vi "test StaticWrite (Func Global).vi"(8 "error in (no error)":errorcluster, 11 "TestCase in":refnum<class "Interface Framework Multiple Objects.lvclass">) -> (0 "error out":errorcluster, 3 "TestCase out":refnum<class "Interface Framework Multiple Objects.lvclass">)   [LabVIEW 2009, in "Interface Framework Multiple Objects.lvclass"]
uses:
  Interface Framework Multiple Objects.lvclass
  Interface Framework Multiple Objects.lvclass/Interface Framework Multiple Objects.ctl
  Numeric Test Object/Interface Implementations/IIntStatic (Func Global)/IIntStatic (Func Global).lvclass
  Numeric Test Object/Numeric Test Object.lvclass
  <vilib>/addons/_JKI Toolkits/VI Tester/TestCase.llb/TestCase.lvclass
  Source/Interfaceable Class/Interfaceable.lvclass
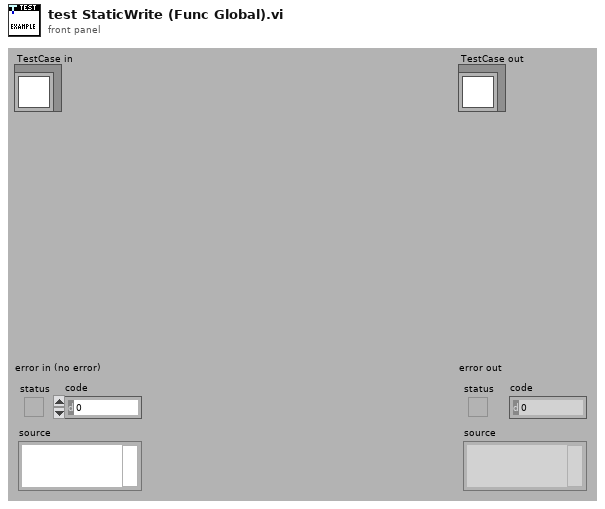
[diagram p1: front panel]
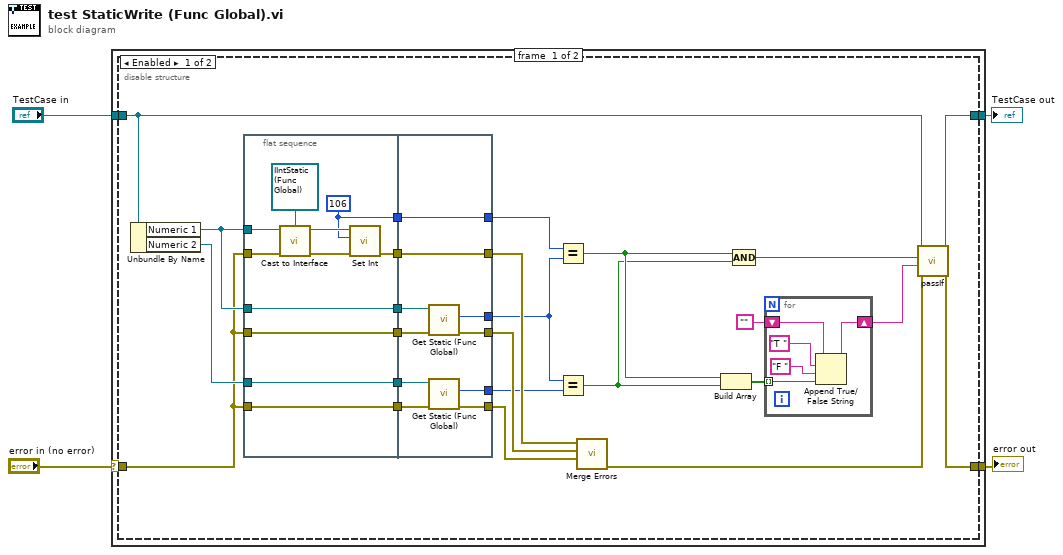
[diagram p0: block diagram]
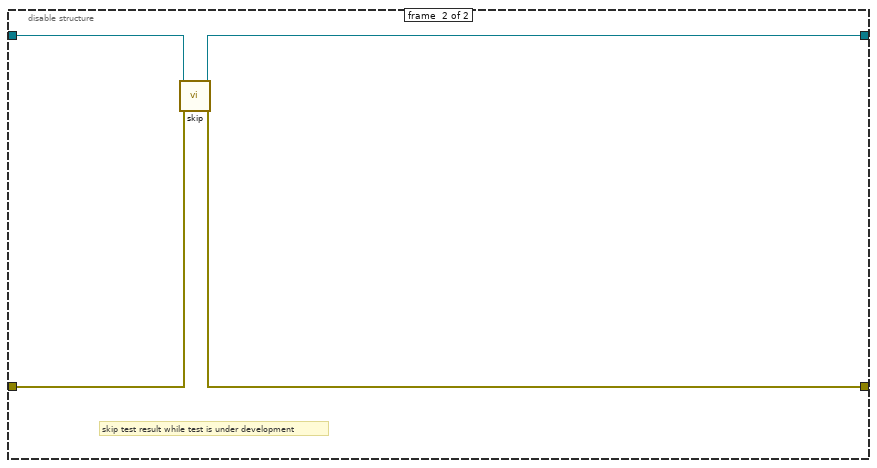
[diagram p2: hidden frame]
diagram:
  n1 = case shown="No Error" "error in (no error)" {
    selector: "error in (no error)" -> [w6 w65]
    tunnel: [w5 w65] -> w3
    tunnel: [w7 w64] -> w1
    tunnel: "TestCase in" -> [w8 w64]
    frame #0 {
      n2 = disable-structure shown="Enabled" {
        disable-tunnel: w8 -> [w31 w63]
        disable-tunnel: [w33 w60] -> w7
        disable-tunnel: w6 -> [w23 w62]
        disable-tunnel: [w32 w61] -> w5
        frame #0 {
          n3 = Unbundle By Name(w31) -> ("Numeric 1"=w29:refnum<class "Numeric Test Object.lvclass">, "Numeric 2"=w30:refnum<class "Numeric Test Object.lvclass">)
          n4 = flat-sequence {
            tunnel: w29 -> [w48]
            tunnel: w30 -> [w41]
            tunnel: w29 -> [w43]
            tunnel: w23 -> [w47]
            tunnel: [w45] -> w28
            tunnel: [w43] -> w27
            tunnel: [w41] -> w26
            tunnel: [w42] -> w25
            tunnel: [w40] -> w24
            tunnel: w23 -> [w40]
            tunnel: w23 -> [w42]
            tunnel: [w39] -> w9
            tunnel: [w51] -> w19
            tunnel: w28 -> [w51]
            tunnel: w27 -> [w59]
            tunnel: w26 -> [w58]
            tunnel: w25 -> [w57]
            tunnel: w24 -> [w56]
            tunnel: [w55] -> w20
            tunnel: [w54] -> w21
            tunnel: [w53] -> w18
            tunnel: [w52] -> w17
            tunnel: [w50] -> w10
            tunnel: w9 -> [w50]
            frame #0 {
              w39 = 106 ("Int")
              n5 = call "Cast to Interface.vi"("Target Interface"=refnum<class "IIntStatic (Func Global).lvclass"> refnum ("IIntByRef.lvclass"), "Interfaceable Object"=w48, "error in (no error)"=w47) -> ("Concrete Interface"=w49:refnum<class "IIntStatic (Func Global).lvclass">, "error out"=w46:errorcluster)  [unwired: 5 in]
              n6 = call-dynamic "Set Int.vi"("error in (no error)"=w46, "Int"=w39, "IIntStatic in"=w49) -> ("error out"=w45:errorcluster)  [unwired: 7 in, 1 out]
            }
            frame #1 {
              n7 = call-dynamic "Get Static (Func Global).vi"("error in (no error)"=w57, "Numeric in"=w59) -> ("error out"=w55:errorcluster, "Int"=w53:i32)  [unwired: 7 in, 1 out]
              n8 = call-dynamic "Get Static (Func Global).vi"("error in (no error)"=w56, "Numeric in"=w58) -> ("error out"=w54:errorcluster, "Int"=w52:i32)  [unwired: 7 in, 1 out]
            }
          }
          n9 = Equal?(x=w10, y=w18) -> (x = y?=w12:bool)
          n10 = Equal?(x=w18, y=w17) -> (x = y?=w11:bool)
          n11 = call <vilib>:"Merge Errors.vi"("error in 3 (no error)"=w21, "error in 2 (no error)"=w20, "error in 1 (no error)"=w19) -> ("error out"=w22:errorcluster)  [unwired: 4 in]
          n12 = Build Array(w12, w11) -> (w15:bool[])
          n13 = Compound Arithmetic op=AND(w12, w11) -> (w14:bool)
          n14 = for {
            tunnel: w15 -> [w38] mode=indexing
            shift-right: [w37] -> w13
            shift-left: "" -> [w34]
            n15 = Append True/False String(1:w38, 2:"F " ("false string"), 3:"T " ("true string"), 4:w34) -> (0:w37:string)
          }
          n16 = call-dynamic "passIf.vi"("error in (no error)"=w22, "message (\"\")"=w13, "pass"=w14, "TestCase in"=w31) -> ("error out"=w32:errorcluster, "TestCase out"=w33:refnum<class "Interface Framework Multiple Objects.lvclass">)  [unwired: 6 in]
        }
        frame #1 {
          # "skip test result while test is under development"
          n17 = call <vilib>:"skip.vi"("error in (no error)"=w62, "TestCase in"=w63) -> ("error out"=w61:errorcluster, "TestCase out"=w60:refnum<class "Interface Framework Multiple Objects.lvclass">)  [unwired: 8 in]
        }
      }
    }
    frame #1 {
    }
  }
  "error out" <- w3
  "TestCase out" <- w1
